vi "CleanUp.vi"(8 "Error In":errorcluster, 11 "object in":refnum<class "ECharts.lvclass">) -> (0 "Error Out":errorcluster, 3 "object out":refnum<class "ECharts.lvclass">)   [LabVIEW 2024, in "ECharts.lvlib" / "ECharts.lvclass"]
uses:
  ECharts.lvclass
  ECharts.lvclass/ECharts.ctl
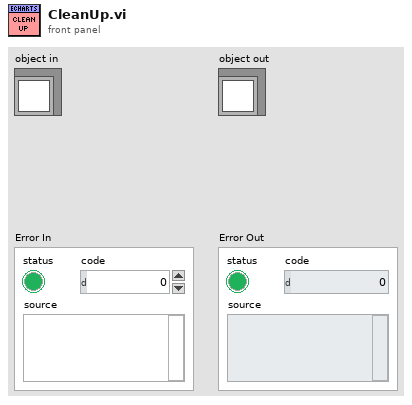
[diagram p1: front panel]
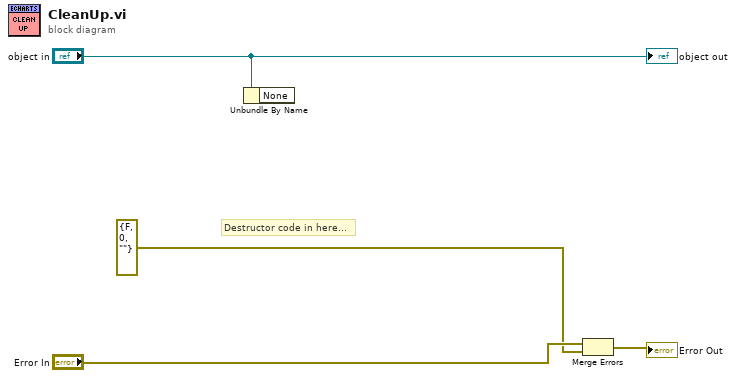
[diagram p0: block diagram]
diagram:
  # "Destructor code in here..."
  n1 = Unbundle By Name("object in") -> ()  [unwired: 1 out]
  n2 = Merge Errors("Error In", errorcluster {"status"=FALSE, "code"=0, "source"=""} ("error in (no error)")) -> (→"Error Out":errorcluster)
  "object out" <- "object in"
